vi "sftpdir.vi"() -> ()   [LabVIEW 2013]
doc: "This example illustrates SFTP directory listing."
uses:
  libssh2/libssh2_init_default.vi
  libssh2/libssh2_session_handshake_tcp.vi
  libssh2/libssh2.lvlib
panel:
  in  "directory":string="/"
  out "individual files":string[](array[string])
  out "directory listing":string
  out "error out":errorcluster
  in  "password":string
  in  "username":string
  in  "hostname":string
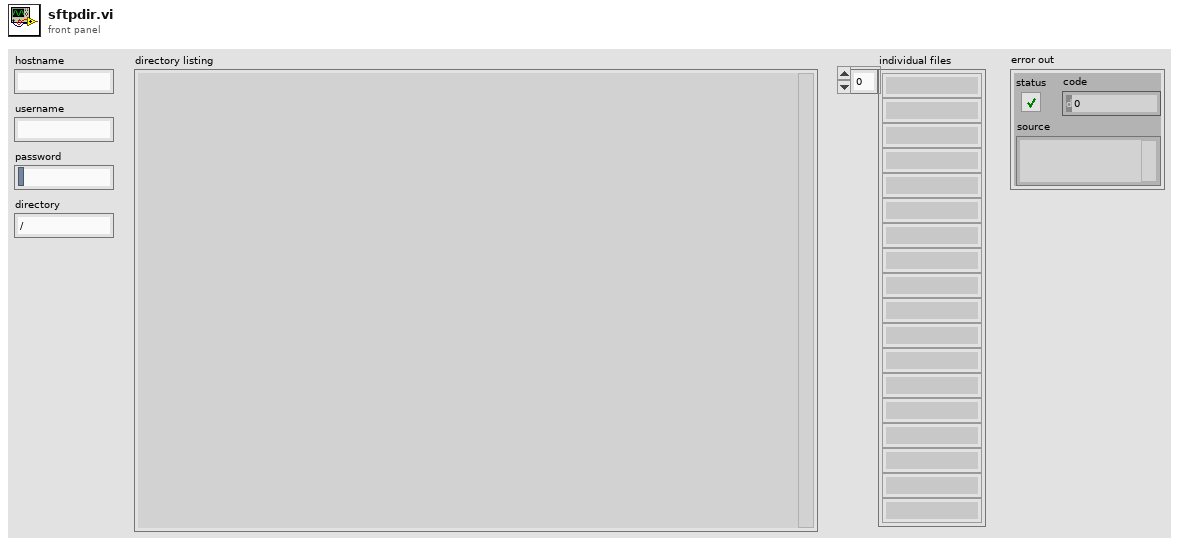
[diagram p1: front panel]
types:
  T1 = typedef "libssh2.lvlib/Session Refnum.ctl" = refnum<k1>
  T2 = typedef "libssh2.lvlib/SFTP Refnum.ctl" = refnum<k1>
  T3 = typedef "libssh2.lvlib/SFTP Handle Refnum.ctl" = refnum<k1>
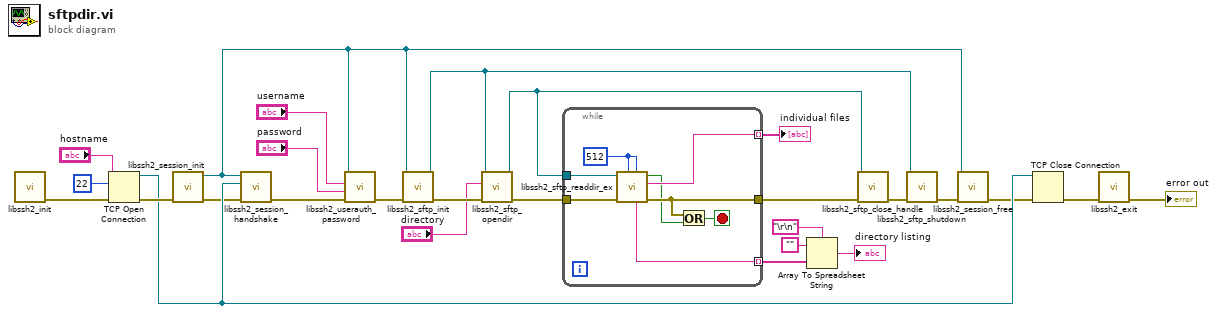
[diagram p0: block diagram]
diagram:
  n1 = call-poly "libssh2_init.vi"() -> ("error out"=w26:errorcluster)  [unwired: 11 in]
  n2 = TCP Open Connection(address="hostname", remote port or service name=u16 22, error in (no error)=w26) -> (connection ID=w24:refnum<k5>, error out=w25:errorcluster)  [unwired: 2 in]
  n3 = call "libssh2_session_init.vi"("error in (no error)"=w25) -> ("error out"=w23:errorcluster, "session"=w16:T1)  [unwired: 9 in]
  n4 = call-poly "libssh2_session_handshake.vi"("error in (no error)"=w23, "tcp connection"=w24, "session"=w16) -> ("error out"=w27:errorcluster)  [unwired: 8 in]
  n5 = call "libssh2_userauth_password.vi"("error in (no error)"=w27, "password"="password", "username"="username", "session"=w16) -> ("error out"=w20:errorcluster)  [unwired: 7 in]
  n6 = call "libssh2_sftp_init.vi"("error in (no error)"=w20, "session"=w16) -> ("error out"=w12:errorcluster, "sftp"=w10:T2)  [unwired: 8 in]
  n7 = call "libssh2_sftp_opendir.vi"("error in (no error)"=w12, "path"="directory", "sftp"=w10) -> ("error out"=w11:errorcluster, "sftp handle"=w6:T3)  [unwired: 7 in]
  n8 = while {
    tunnel: w11 -> [w35]
    tunnel: [w31] -> w7
    tunnel: w6 -> [w34]
    tunnel: [w28] -> w4 mode=indexing
    tunnel: [w32] -> w1 mode=indexing
    stop <- w29 stop-if-true
    w33 = 512 ("buffer maxlen")
    n9 = call "libssh2_sftp_readdir_ex.vi"("longentry maxlen (0)"=w33, "buffer maxlen"=w33, "error in (no error)"=w35, "sftp handle"=w34) -> ("error out"=w31:errorcluster, "buffer"=w32:string, "no more files"=w30:bool, "longentry"=w28:string)  [unwired: 3 in, 1 out]
    n10 = Or(x=w31, y=w30) -> (x .or. y?=w29:bool)
  }
  "individual files" <- w1
  n11 = Array To Spreadsheet String(delimiter (Tab)="\r\n", array=w4, 3:"" ("format string")) -> (spreadsheet string=→"directory listing":string)
  n12 = call "libssh2_sftp_close_handle.vi"("error in (no error)"=w7, "sftp handle"=w6) -> ("error out"=w8:errorcluster)  [unwired: 9 in]
  n13 = call "libssh2_sftp_shutdown.vi"("error in (no error)"=w8, "sftp"=w10) -> ("error out"=w13:errorcluster)  [unwired: 9 in]
  n14 = call "libssh2_session_free.vi"("error in (no error)"=w13, "session"=w16) -> ("error out"=w15:errorcluster)  [unwired: 9 in]
  n15 = TCP Close Connection(connection ID=w24, error in (no error)=w15) -> (error out=w14:errorcluster)  [unwired: 1 in, 1 out]
  n16 = call "libssh2_exit.vi"("error in (no error)"=w14) -> ("error out"=→"error out":errorcluster)  [unwired: 10 in]
